vi "Measurement Logic.vi"(8 "error in":errorcluster, 10 "measure call context in":refnum<class "Measure Call Context.lvclass">, 11 "measurement configuration":T2={"Input channel"=0, "Full scale range"=10.0, "Analog source resource name"="", "Analog source sample rate"=800000.0, "Ramp samples"=800000, "Ramp start"=1000.0, "Ramp stop"=-1.0, "Digital capture resource name"="", "Digital capture sample rate"=800000.0, "Digital capture samples"=800000, "DMM resource name"="", "DMM range"=800000.0, "DMM resolution"=800000.0}) -> (0 "error out":errorcluster, 2 "measure call context out":refnum<class "Measure Call Context.lvclass">)   [LabVIEW 2021, in "Gain And Offset_ADC.lvlib"]
uses:
  Gain And Offset_ADC.lvlib
  Measurement Configuration.ctl
  <vilib>/MeasurementLink/MeasurementLink Measurement Server/Measure Call Context/Measure Call Context.lvclass
  Measurement Results.ctl
  <vilib>/gRPC/LabVIEW gRPC Library/Shared/grpcId.ctl
  <instrlib>/niDMM/nidmm.llb/niDMM Function.ctl
  <vilib>/DAQmx/create/channels.llb/DAQmx Create Channel (AO-Voltage-Basic).vi
  <vilib>/DAQmx/configure/timing.llb/DAQmx Timing (Sample Clock).vi
  <instrlib>/niDMM/nidmm.llb/niDMM Configure Measurement Digits.vi
  shared/digitalInterface/client/dcvmDPI_AD7606B_client/dcvmDPI_AD7606B_client.lvlib
  <vilib>/gRPC/LabVIEW gRPC Library/grpc-lvsupport-release.lvlib
  shared/digitalInterface/client/dcvmDPI_AD7606B_clientImpl/dcvmDPI_AD7606B_clientImpl.lvlib
panel:
  out "measurement results":T1
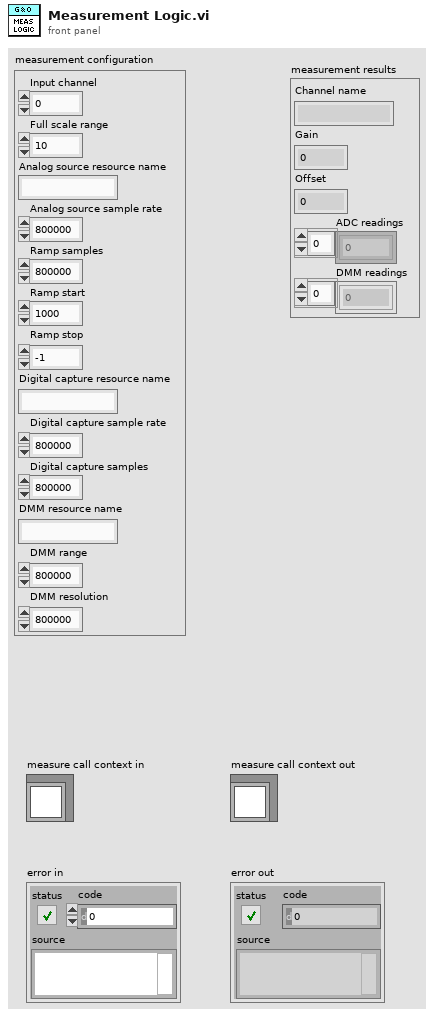
[diagram p1: front panel]
types:
  T1 = typedef "Gain And Offset_ADC.lvlib/Measurement Results.ctl" = cluster{"Channel name":string, "Gain":dbl, "Offset":dbl, "ADC readings":dbl[], "DMM readings":dbl[]}
  T2 = typedef "Gain And Offset_ADC.lvlib/Measurement Configuration.ctl" = cluster{"Input channel":i32, "Full scale range":dbl, "Analog source resource name":string, "Analog source sample rate":dbl, "Ramp samples":i32, "Ramp start":dbl, "Ramp stop":dbl, "Digital capture resource name":string, "Digital capture sample rate":dbl, "Digital capture samples":u32, "DMM resource name":string, "DMM range":dbl, "DMM resolution":dbl}
  T3 = typedef "grpc-lvsupport-release.lvlib/grpcId.ctl" = u64
  T4 = cluster{"DSG Session":refnum<k21>, "DMM Session":refnum<k15>, "gRPC session":T3}
  T5 = typedef "niDMM Function.ctl" = enum16{"DC Volts", "AC Volts", "DC Current", "AC Current", "2-wire Resistance", "4-wire Resistance", "Diode", "Frequency", "Period", "AC Volts DC Coupled", "Capacitance", "Inductance", "Temperature"}
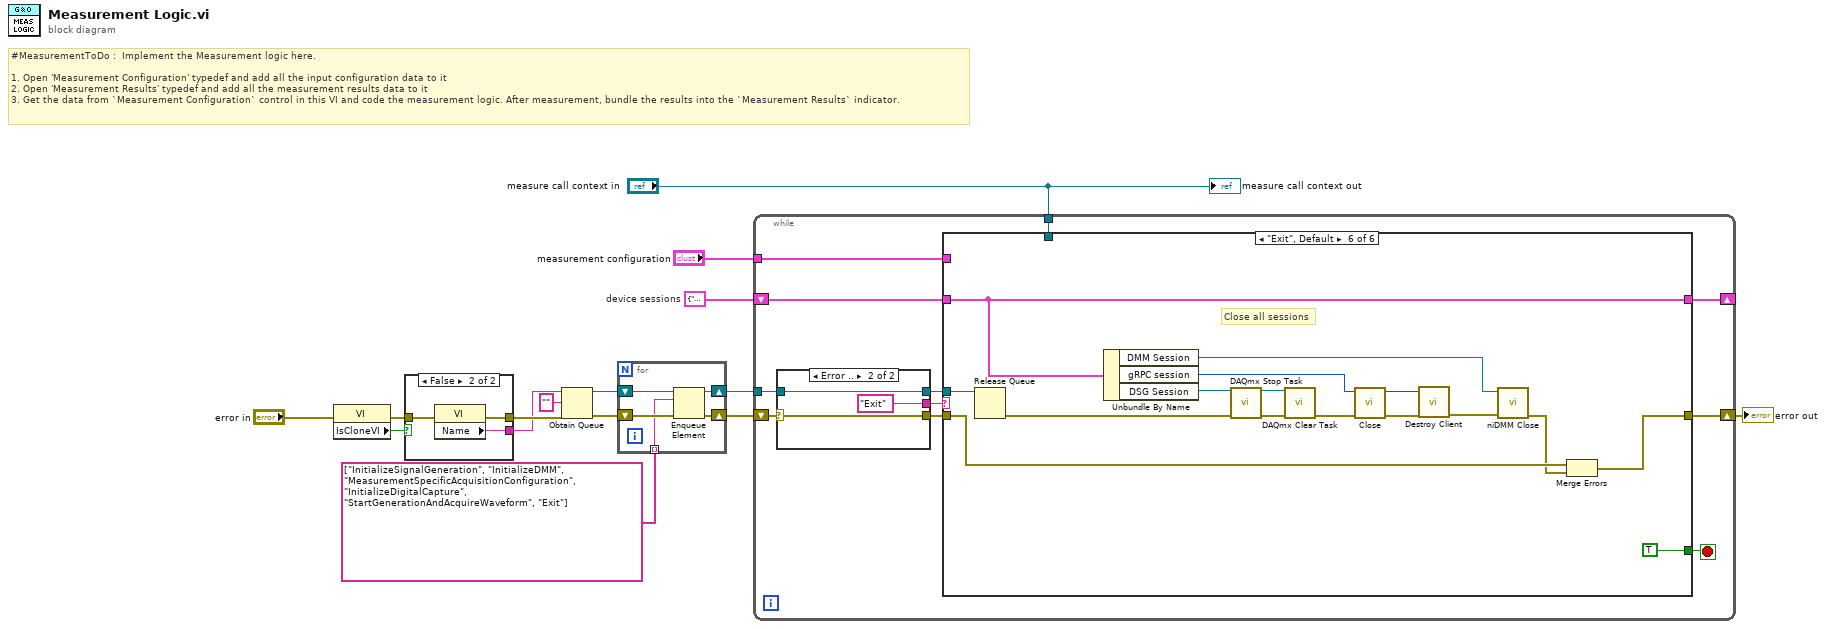
[diagram p0: block diagram]
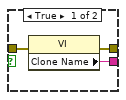
[diagram p2: hidden frame]
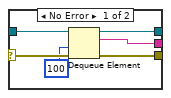
[diagram p3: hidden frame]
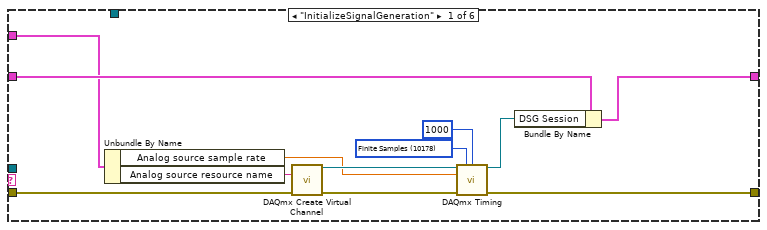
[diagram p4: hidden frame]
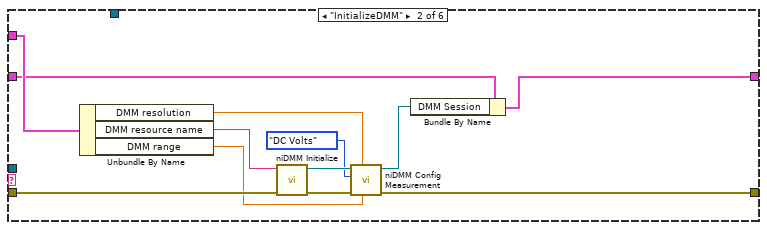
[diagram p5: hidden frame]
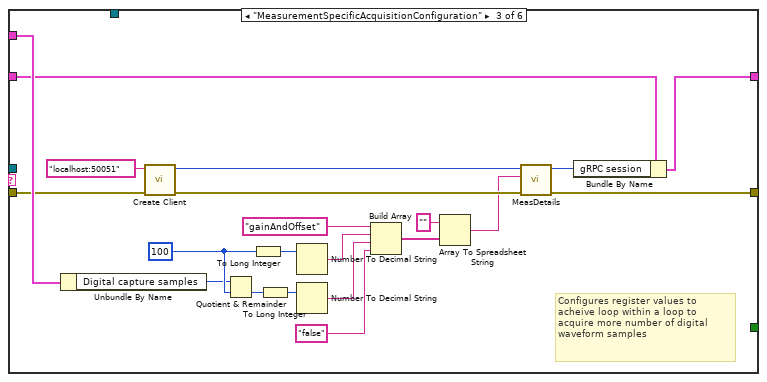
[diagram p6: hidden frame]
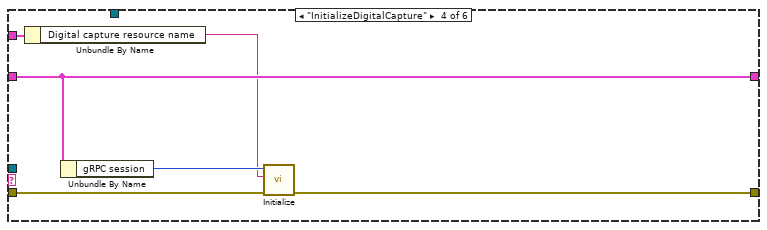
[diagram p7: hidden frame]
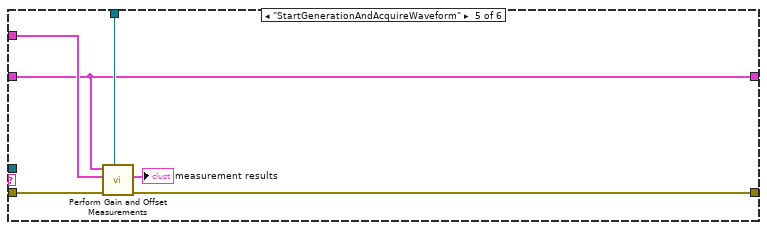
[diagram p8: hidden frame]
diagram:
  w12 = T4 {"DSG Session"="", "DMM Session"="", "gRPC session"=0}  # device sessions
  # "#MeasurementToDo :  Implement the Measurement logic here.\n\n1. Open 'Measurement Configuration' typedef and add all the input configuration data to it\n2. Open 'Measurement Results' typedef and add all the measurement results data to it\n3. Get the data from `Measurement Configuration` control in this VI and code the measurement logic. After measurement, bundle the results into the `Measurement Results` indicator."
  n1 = property class="VI"(error in="error in") -> (error out=w7:errorcluster, "IsCloneVI"=w8:bool)  [unwired: 1 in, 1 out]
  n2 = case shown="False" w8 {
    tunnel: [w18 w21] -> w5
    tunnel: [w17 w20] -> w4
    tunnel: w7 -> [w16 w19]
    frame True {
      n3 = property class="VI"(error in=w16) -> (error out=w18:errorcluster, "Clone Name"=w17:string)  [unwired: 1 in, 1 out]
    }
    frame False {
      n4 = property class="VI"(error in=w19) -> (error out=w21:errorcluster, "Name"=w20:string)  [unwired: 1 in, 1 out]
    }
  }
  n5 = Obtain Queue(name (unnamed)=w4, element data type="", error in (no error)=w5) -> (queue out=w14:refnum<queue>, error out=w3:errorcluster)  [unwired: 2 in, 1 out]
  n6 = for {
    shift-right: [w24] -> w13
    shift-left: w14 -> [w26]
    shift-right: [w23] -> w2
    shift-left: w3 -> [w25]
    tunnel: string[] ["InitializeSignalGeneration", "InitializeDMM", "MeasurementSpecificAcquisitionConfiguration", "InitializeDigitalCapture", "StartGenerationAndAcquireWaveform", "Exit"] ("Step sequence") -> [w22] mode=indexing
    n7 = Enqueue Element(queue=w26, element=w22, error in (no error)=w25) -> (queue out=w24:refnum<queue>, error out=w23:errorcluster)  [unwired: 1 in, 1 out]
  }
  n8 = while {
    tunnel: w13 -> [w31]
    shift-right: [w37] -> w9
    shift-left: w2 -> [w32]
    tunnel: "measurement configuration" -> [w35]
    shift-right: [w33] -> _
    shift-left: w12 -> [w34]
    tunnel: "measure call context in" -> [w27]
    stop <- w36 stop-if-true
    n9 = case shown="Error .." w32 {
      selector: w32 -> [w41 w45]
      tunnel: w31 -> [w43 w44]
      tunnel: [w42 "Exit" ("t")] -> w30
      tunnel: [w40 w45] -> w29
      tunnel: [w38 w44] -> w28
      frame No Error {
        n10 = Dequeue Element(queue=w43, timeout in ms (-1)=100, error in (no error)=w41) -> (queue out=w38:refnum<queue>, element=w42:string, error out=w40:errorcluster)  [unwired: 1 out]
      }
      frame Error {
      }
    }
    n11 = case shown="\"Exit\", Default" w30 {
      tunnel: [w56 w62 w71 w92 w103 w111] -> w37
      tunnel: w29 -> [w57 w68 w87 w96 w100 w112]
      tunnel: [_ _ _ _ _ TRUE] -> w36
      tunnel: w35 -> [w53 w70 w90 w97 w102 _]
      tunnel: w34 -> [w55 w61 w74 w95 w98 w115]
      tunnel: [w54 w59 w72 w95 w98 w115] -> w33
      tunnel: w28 -> [_ _ _ _ _ w114]
      tunnel: w27 -> [_ _ _ _ w99 _]
      frame "InitializeSignalGeneration" {
        w49 = 10178 items=["Finite Samples"=10178, "Continuous Samples"=10123, "Hardware Timed Single Point"=12522] ("sample mode")
        n12 = Unbundle By Name(w53) -> ("Analog source sample rate"=w47:dbl, "Analog source resource name"=w58:string)
        n13 = call-poly <vilib>:"DAQmx Create Virtual Channel.vi"("physical channels"=w58, "error in"=w57) -> ("task out"=w51:refnum<k21>, "error out"=w50:errorcluster)  [unwired: 12 in]
        n14 = call-poly <vilib>:"DAQmx Timing.vi"("task/channels in"=w51, "sample mode"=w49, "samples per channel"=1000, "rate"=w47, "error in"=w50) -> ("task out"=w52:refnum<k21>, "error out"=w56:errorcluster)  [unwired: 9 in]
        n15 = Bundle By Name(cluster=w55, "DSG Session"=w52) -> (w54:T4)
      }
      frame "InitializeDMM" {
        n16 = Unbundle By Name(w70) -> ("DMM resolution"=w65:dbl, "DMM resource name"=w69:string, "DMM range"=w64:dbl)
        n17 = call <instrlib>:"niDMM Initialize.vi"("error in (no error)"=w68, "Instrument Descriptor"=w69) -> ("error out"=w67:errorcluster, "instrument handle out"=w66:refnum<k15>)  [unwired: 8 in]
        n18 = call-poly <instrlib>:"niDMM Config Measurement.vi"("Range"=w64, "Resolution in Digits"=w65, "error in (no error)"=w67, "Function"=niDMM_Function."DC Volts", "instrument handle"=w66) -> ("error out"=w62:errorcluster, "instrument handle out"=w60:refnum<k15>)  [unwired: 5 in]
        n19 = Bundle By Name(cluster=w61, "DMM Session"=w60) -> (w59:T4)
      }
      frame "MeasurementSpecificAcquisitionConfiguration" {
        w91 = u32 100 ("value")
        # "Configures register values to acheive loop within a loop to acquire more number of digital waveform samples"
        n20 = Unbundle By Name(w90) -> ("Digital capture samples"=w89:u32)
        n21 = call "Create Client.vi"("error in"=w87, "address"="localhost:50051") -> ("error out"=w77:errorcluster, "gRPC ID Out"=w76:T3)  [unwired: 8 in]
        n22 = Quotient & Remainder(x=w89, y=w91) -> (floor(x/y)=w88:u32)  [unwired: 1 out]
        n23 = To Long Integer(number=w91) -> (32bit integer=w85:i32)
        n24 = To Long Integer(number=w88) -> (32bit integer=w84:i32)
        n25 = Number To Decimal String(number=w85) -> (decimal integer string=w82:string)  [unwired: 1 in]
        n26 = Number To Decimal String(number=w84) -> (decimal integer string=w81:string)  [unwired: 1 in]
        n27 = Build Array("gainAndOffset", w82, w81, "false") -> (w79:string[])
        n28 = Array To Spreadsheet String(array=w79, 3:"" ("format string")) -> (spreadsheet string=w75:string)  [unwired: 1 in]
        n29 = call "MeasDetails.vi"("error in"=w77, "Active measurement"=w75, "gRPC session in"=w76) -> ("error out"=w71:errorcluster, "gRPC session out"=w73:T3)  [unwired: 7 in]
        n30 = Bundle By Name(cluster=w74, "gRPC session"=w73) -> (w72:T4)
      }
      frame "InitializeDigitalCapture" {
        n31 = Unbundle By Name(w97) -> ("Digital capture resource name"=w93:string)
        n32 = Unbundle By Name(w95) -> ("gRPC session"=w94:T3)
        n33 = call "Initialize.vi"("error in"=w96, "Digital capture resource name"=w93, "gRPC session in"=w94) -> ("error out"=w92:errorcluster)  [unwired: 7 in, 1 out]
      }
      frame "StartGenerationAndAcquireWaveform" {
        n34 = call "Perform Gain and Offset Measurements.vi"("Measurement Context"=w99, "error in"=w100, "measurement configuration"=w102, "device sessions"=w98) -> ("error out"=w103:errorcluster, "measurement results"=→"measurement results":T1)  [unwired: 6 in]
      }
      frame "Exit", Default {
        # "Close all sessions"
        n35 = Release Queue(queue=w114) -> (error out=w113:errorcluster)  [unwired: 2 in, 2 out]
        n36 = Unbundle By Name(w115) -> ("DMM Session"=w109:refnum<k15>, "gRPC session"=w108:T3, "DSG Session"=w118:refnum<k21>)
        n37 = call <vilib>:"DAQmx Stop Task.vi"("task/channels in"=w118, "error in"=w113) -> ("task out"=w117:refnum<k21>, "error out"=w116:errorcluster)  [unwired: 12 in]
        n38 = call <vilib>:"DAQmx Clear Task.vi"("task in"=w117, "error in"=w116) -> ("error out"=w107:errorcluster)  [unwired: 13 in]
        n39 = call "Close.vi"("error in"=w107, "gRPC session in"=w108) -> ("error out"=w105:errorcluster, "gRPC session out"=w106:T3)  [unwired: 8 in]
        n40 = call "Destroy Client.vi"("error in"=w105, "gRPC ID"=w106) -> ("error out"=w104:errorcluster)  [unwired: 9 in]
        n41 = call <instrlib>:"niDMM Close.vi"("error in (no error)"=w104, "instrument handle"=w109) -> ("error out"=w110:errorcluster)  [unwired: 9 in]
        n42 = Merge Errors(w112, w110) -> (w111:errorcluster)
      }
    }
  }
  "error out" <- w9
  "measure call context out" <- "measure call context in"
